vi "cut_img.vi"() -> ()   [LabVIEW 2015]
uses:
  <vilib>/picture/picture.llb/Draw True-Color Pixmap.vi
panel:
  in  "Unde? 2":path
  out "new picture":picture
  in  "Care Imagine?":path
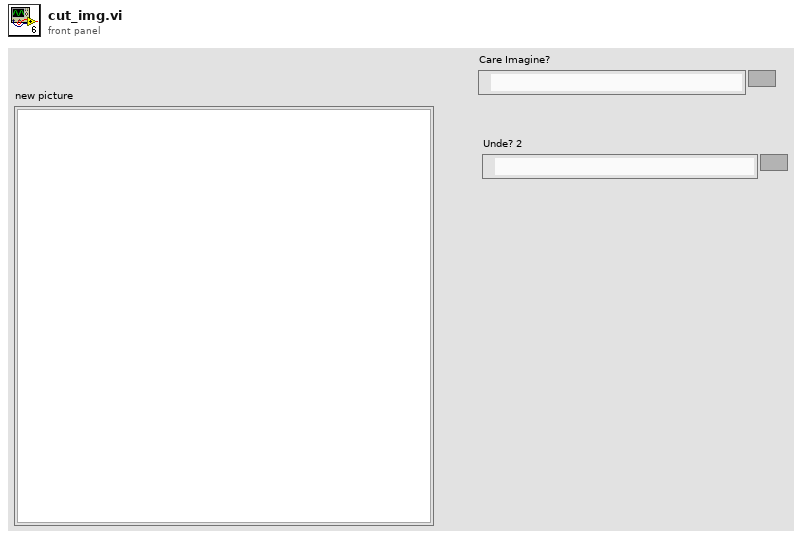
[diagram p1: front panel]
types:
  T1 = typedef "imagedata.ctl" = cluster{"image type":i32, "image depth":i32, "image":u8[], "mask":u8[], "colors":u32[], "Rectangle":cluster{"left":i16, "top":i16, "right":i16, "bottom":i16}}
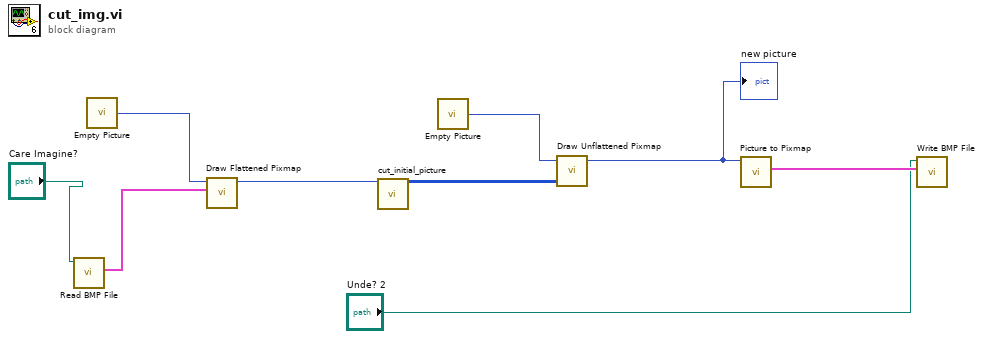
[diagram p0: block diagram]
diagram:
  n1 = call <vilib>:"Read BMP File.vi"("path to BMP file"="Care Imagine?") -> ("image data"=w1:T1)  [unwired: 8 in, 2 out]
  n2 = call "Empty Picture"() -> ("empty picture"=w9:picture)
  n3 = call <vilib>:"Draw Flattened Pixmap.vi"("image data"=w1, "picture"=w9) -> ("new picture"=w8:picture)  [unwired: 7 in]
  n4 = call "cut_initial_picture.vi"("picture"=w8) -> ("new"=w7:u32[][])  [unwired: 14 in]
  n5 = call "Empty Picture"() -> ("empty picture"=w6:picture)
  n6 = call-poly <vilib>:"Draw Unflattened Pixmap.vi"("picture"=w6, "data (RGB format)"=w7) -> ("new picture"=w5:picture)  [unwired: 7 in]
  "new picture" <- w5
  n7 = call <vilib>:"Picture to Pixmap.vi"("picture"=w5) -> ("image data"=w4:T1)  [unwired: 9 in, 1 out]
  n8 = call <vilib>:"Write BMP File.vi"("image data"=w4, "path to BMP file"="Unde? 2") -> ()  [unwired: 8 in, 2 out]
